vi "Butterfly_PullDown Capacitance _ERMod.vi"(0 "Semiconductor Module Context":T2, 1 "Capacitance":bool=TRUE, 3 "RFPins":string[](array[string]), 4 "VNAs Measurement Parameters":T1, 5 "error in (no error)":errorcluster, 7 "C_TH_Delta":dbl=2.0, 8 "R Thresholds":dbl[](array[numeric]), 9 "Start_v":dbl=10.0 format="%#_13g", 11 "Stop_v":dbl=41.0 format="%#_13g") -> (14 "Semiconductor Module Context Out":T2, 19 "error out":errorcluster)   [LabVIEW 2013]
uses:
  <vilib>/NI_TestStand_SemiconductorModule/NI_TestStand_Semiconductor_Module.lvlibp/PinMap/General/SemiconductorModuleContext.ctl
  VNA/VNAs Measurement Parameters.ctl
  <instrlib>/niDCPower/nidcpower.llb/niDCPower Wait For Event - Event.ctl
  <vilib>/NI_TestStand_SemiconductorModule/NI_TestStand_Semiconductor_Module.lvlibp/PinMap/DC Power/PinsToNIDCPowerSessions.vi
  <vilib>/NI_TestStand_SemiconductorModule/NI_TestStand_Semiconductor_Module.lvlibp/PinMap/General/Publish/PublishDataDoubleFunctionalTest.vi
  <vilib>/NI_TestStand_SemiconductorModule/NI_TestStand_Semiconductor_Module.lvlibp/PinMap/General/Publish/PublishDataDouble2D.vi
  <vilib>/NI_TestStand_SemiconductorModule/NI_TestStand_Semiconductor_Module.lvlibp
  VNA/Pin Map API/VNA Custom Instrument.lvlib
panel:
  out "C_Free":dbl[](array[numeric])
  out "VRLs":dbl[][](array[numeric]) format="%#_3g"
  out "VPIs":dbl[][](array[numeric]) format="%#_3g"
  out "appended array":dbl[][](array[numeric]) format="%#_3g"
  out "S3 steps":dbl[](array[numeric]) format="%#_3g"
  out "S2 steps":dbl[](array[numeric]) format="%#_3g"
  out "S1 steps":dbl[](array[numeric]) format="%#_3g"
  out "S0 steps":dbl[](array[numeric]) format="%#_3g"
  out "BF values":dbl[](array[numeric])
  out "VRLs":dbl[](array[numeric])
  out "VPIs":dbl[](array[numeric])
  out "Multisite Cap Data":dbl[][][](array[numeric])
  out "Full Array":dbl[][][](array[numeric])
  out "BF Names":string[](array[string])
  in  "current level":dbl=0.01 format="%_6p"
  out "R Array":dbl[](array[numeric])
  out "BFSamples":i32
  in  "Step_v":dbl=1.0
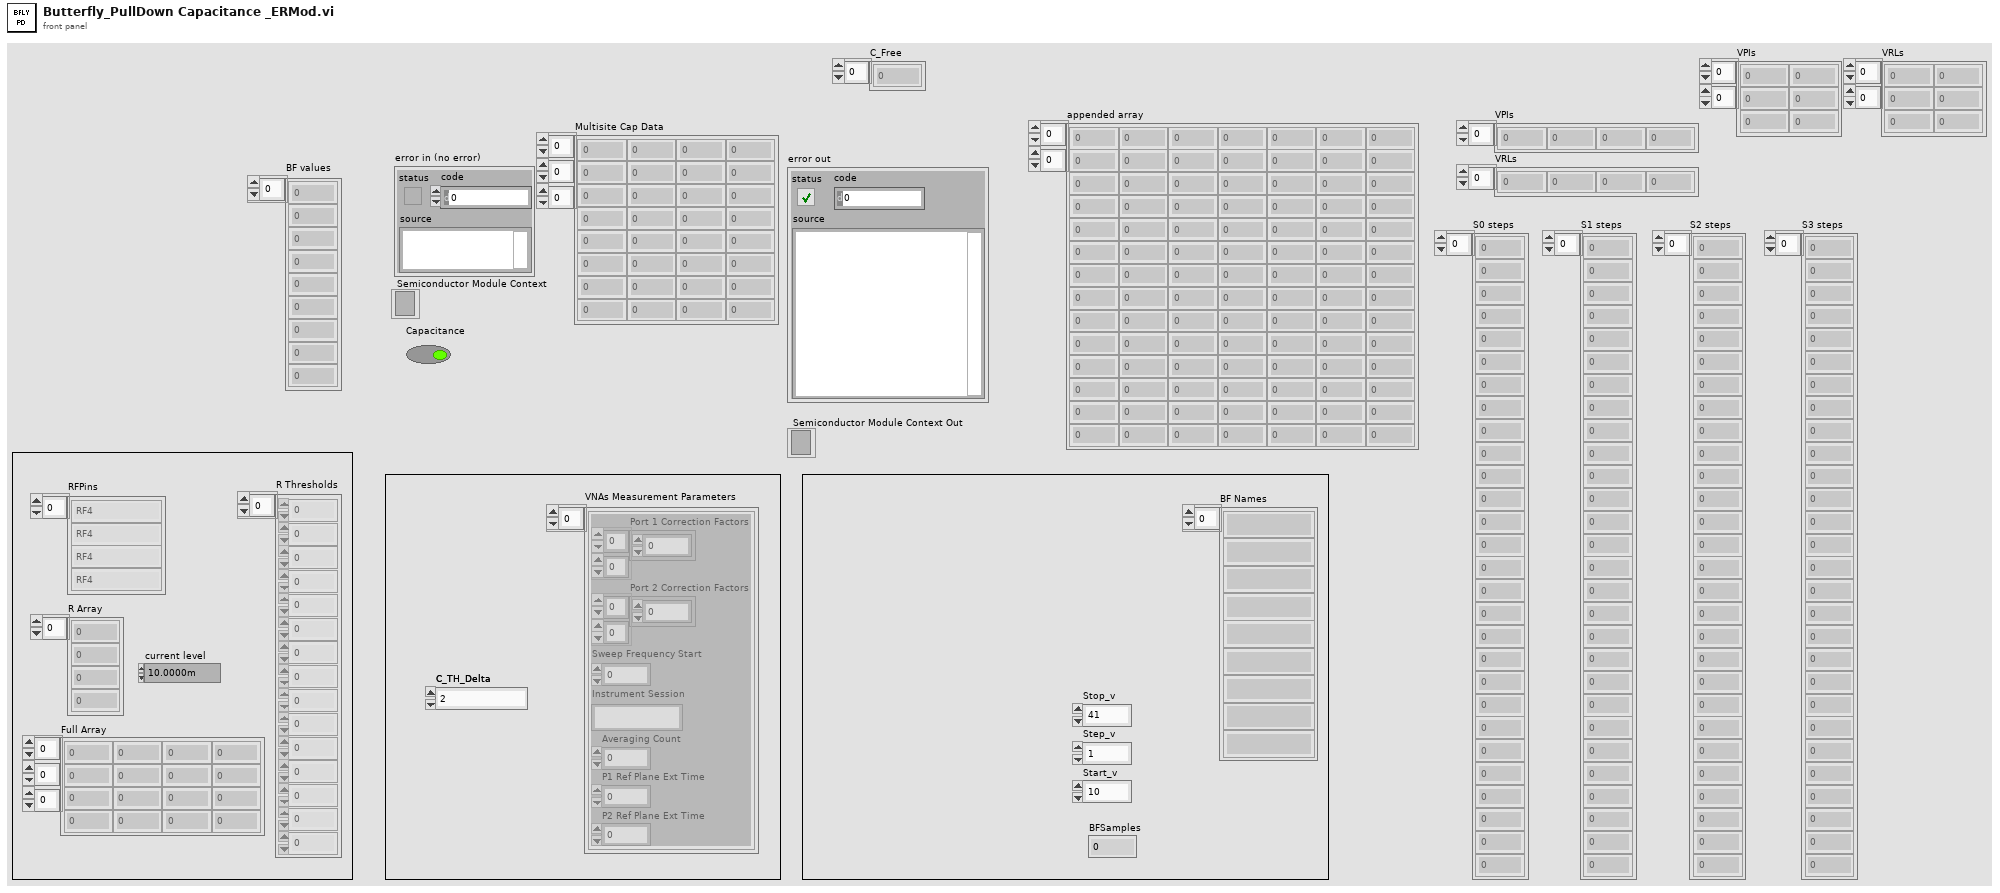
[diagram p1: front panel]
types:
  T1 = typedef "VNAs Measurement Parameters.ctl" = cluster{"Port 1 Correction Factors":cdb[][], "Port 2 Correction Factors":cdb[][], "Sweep Frequency Start":dbl, "Instrument Session":string, "Averaging Count":i32, "P1 Ref Plane Ext Time":dbl, "P2 Ref Plane Ext Time":dbl}[]
  T2 = typedef "NI_TestStand_Semiconductor_Module.lvlibp/SemiconductorModuleContext.ctl" = refnum<k7>
  T3 = typedef "niDCPower Wait For Event - Event.ctl" = i32
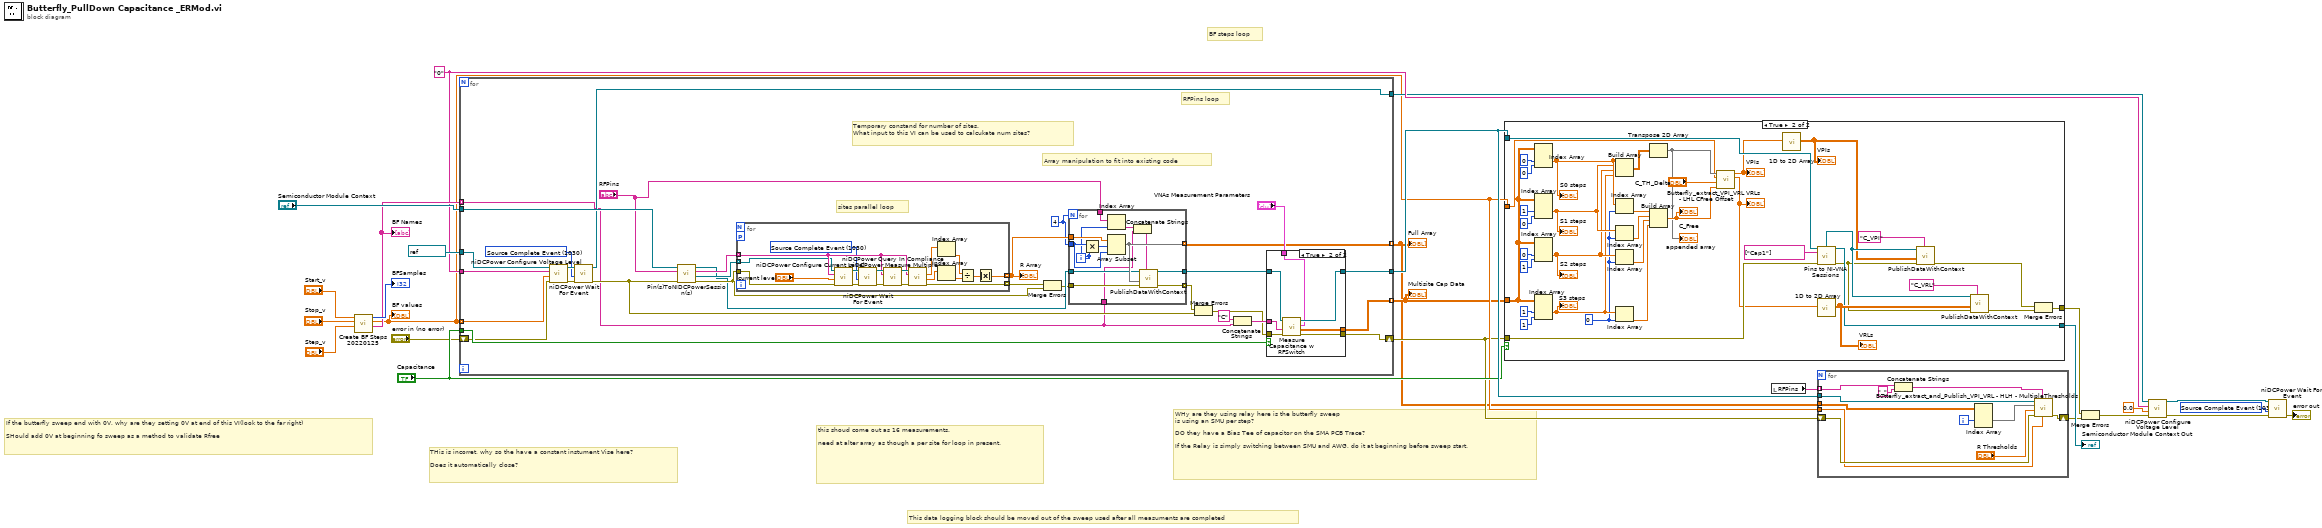
[diagram p0: block diagram]
diagram:
  w8 = T3 1030 items=["Source Complete Event"=1030, "Measure Complete Event"=1031, "Sequence Iteration Complete Event"=1032, "Sequence Engine Done Event"=1033, "Pulse Complete Event"=1051, "Ready For Pulse Trigger Event"=1052] ("event")
  w13 = "0" ("channel name")
  # "If the butterfly sweep end with 0V, why are they setting 0V at end of this VI(look to the far right)\n\nSHould add 0V at beginning fo sweep as a method to validate Rfree"
  # "This data logging block should be moved out of the sweep used after all measuments are completed"
  # "THis is incorret, why so the have a constant instument Vise here?\n\nDoes it automatically close?"
  # "WHy are they using relay here is the butterfly sweep \nis using an SMU per step?\n\nDO they have a Bias Tee of capacitor on the SMA PCB Trace?\n\nIf the Relay is simply switching between SMU and AWG, do it at beginning before sweep start."
  # "this shoud come out as 16 measurements. \n\nneed at alter array as though a per site for loop in present."
  # "BF steps loop"
  n1 = call "Create BF Steps 20220125.vi"("Step_v"="Step_v", "Stop_v"="Stop_v", "Start_v"="Start_v") -> ("BF Names"=w17:string[], "BF values"=w7:dbl[], "BFSamples"=→"BFSamples":i32)  [unwired: 6 in]
  "BF Names" <- w17
  "BF values" <- w7
  n2 = for {
    shift-right: [w40] -> w5
    shift-left: "error in (no error)" -> [w46]
    tunnel: "Semiconductor Module Context" -> [w57]
    tunnel: [w56] -> w23
    tunnel: [w52] -> w6 mode=indexing
    tunnel: "Capacitance" -> [w50]
    tunnel: w17 -> [w27] mode=indexing
    tunnel: w7 -> [w44] mode=indexing
    tunnel: w13 -> [w43]
    tunnel: refnum<k15> "4139_1" ("instrument handle") -> [w42]
    tunnel: [w41] -> w12
    tunnel: [w33] -> w1 mode=indexing
    w34 = 4
    w48 = T3 1030 items=["Source Complete Event"=1030, "Measure Complete Event"=1031, "Sequence Iteration Complete Event"=1032, "Sequence Engine Done Event"=1033, "Pulse Complete Event"=1051, "Ready For Pulse Trigger Event"=1052] ("event")
    # "Array manipulation to fit into existing code"
    # "Temporary constand for number of sites.\nWhat input to this VI can be used to calcukate num sites?"
    # "sites parallel loop"
    # "RFPins loop"
    n3 = call <instrlib>:"niDCPower Configure Voltage Level.vi"("error in (no error)"=w46, "voltage level"=w44, "channel name"=w43, "instrument handle"=w42) -> ("error out"=w47:errorcluster, "instrument handle out"=w49:refnum<k15>)  [unwired: 6 in]
    n4 = call <instrlib>:"niDCPower Wait For Event.vi"("error in (no error)"=w47, "event"=w48, "instrument handle"=w49) -> ("error out"=w45:errorcluster, "instrument handle out"=w41:refnum<k15>)  [unwired: 7 in]
    n5 = call-poly <vilib>:"Pin(s)ToNIDCPowerSession(s).vi"("error in (no error)"=w45, "Pins"="RFPins", "Semiconductor Module Context"=w57) -> ("error out"=w37:errorcluster, "Instrument Sessions"=w38:refnum<k15>[], "Channel Lists"=w39:string[], "Semiconductor Module Context Out"=w32:T2)  [unwired: 4 in, 1 out]
    n6 = for {
      tunnel: w39 -> [w75] mode=indexing
      tunnel: w38 -> [w71] mode=indexing
      tunnel: w37 -> [w72]
      tunnel: [w76] -> w35 mode=indexing
      workers-P: _ -> [_]
      tunnel: [w73] -> w36 mode=indexing
      w74 = T3 1030 items=["Source Complete Event"=1030, "Measure Complete Event"=1031, "Sequence Iteration Complete Event"=1032, "Sequence Engine Done Event"=1033, "Pulse Complete Event"=1051, "Ready For Pulse Trigger Event"=1052] ("event")
      n7 = call <instrlib>:"niDCPower Configure Current Level.vi"("error in (no error)"=w72, "current level"="current level", "channel name"=w75, "instrument handle"=w71) -> ("error out"=w84:errorcluster, "instrument handle out"=w83:refnum<k15>)  [unwired: 6 in]
      n8 = call <instrlib>:"niDCPower Wait For Event.vi"("error in (no error)"=w84, "event"=w74, "instrument handle"=w83) -> ("error out"=w88:errorcluster, "instrument handle out"=w87:refnum<k15>)  [unwired: 7 in]
      n9 = call <instrlib>:"niDCPower Query In Compliance.vi"("error in (no error)"=w88, "channel name"=w75, "instrument handle"=w87) -> ("error out"=w85:errorcluster, "instrument handle out"=w86:refnum<k15>)  [unwired: 6 in, 1 out]
      n10 = call <instrlib>:"niDCPower Measure Multiple.vi"("error in (no error)"=w85, "channel name"=w75, "instrument handle"=w86) -> ("error out"=w73:errorcluster, "current measurements"=w77:dbl[], "voltage measurements"=w78:dbl[])  [unwired: 5 in, 1 out]
      n11 = Index Array(array=w78) -> (element=w80:dbl)  [unwired: 1 in]
      n12 = Index Array(array=w77) -> (element=w79:dbl)  [unwired: 1 in]
      n13 = Divide(x=w80, y=w79) -> (x/y=w81:dbl)
      n14 = Absolute Value(x=w81) -> (abs(x)=w76:dbl)
    }
    "R Array" <- w35
    n15 = Merge Errors(w36, w37) -> (w30:errorcluster)
    n16 = for {
      N: w34 -> [_]
      tunnel: w35 -> [w70]
      tunnel: w34 -> [w69]
      tunnel: [w67] -> w33 mode=indexing
      tunnel: w32 -> [w66]
      tunnel: [w65] -> w31
      tunnel: w30 -> [w64]
      tunnel: [w63] -> w29 mode=indexing
      tunnel: "RFPins" -> [w62]
      tunnel: w27 -> [w60]
      i -> [w61]
      n17 = Multiply(x=w69, y=w61) -> (x*y=w68:i32)
      n18 = Array Subset(array=w70, index=w68, length=w69) -> (w67:dbl[])
      n19 = Index Array(array=w62, index=w61) -> (element=w59:string)
      n20 = Concatenate Strings(w59, w60) -> (w58:string)
      n21 = call-poly <vilib>:"PublishDataWithContext.vi"("Published Data Id"=w58, "error in (no error)"=w64, "Data In"=w67, "Semiconductor Module Context"=w66) -> ("error out"=w63:errorcluster, "Semiconductor Module Context Out"=w65:T2)  [unwired: 6 in]
    }
    n22 = Merge Errors(w29, w45) -> (w51:errorcluster)
    n23 = Concatenate Strings("C" ("string"), w27) -> (w54:string)
    n24 = case shown="True" w50 {
      tunnel: w31 -> [w90 w97]
      tunnel: [w90 w96] -> w56
      tunnel: [w89 w95] -> w40
      tunnel: w54 -> [_ w94]
      tunnel: "VNAs Measurement Parameters" -> [_ w93]
      tunnel: [_ w92] -> w52
      tunnel: w51 -> [w89 w91]
      frame False {
      }
      frame True {
        n25 = call "Measure Capacitance w RFSwitch.vi"("VNAs Measurement Parameters"=w93, "error in (no error)"=w91, "Measurement Id"=w94, "Semiconductor Module Context"=w97) -> ("error out"=w95:errorcluster, "Multisite Cap Data"=w92:dbl[][], "Semiconductor Module Context Out"=w96:T2)  [unwired: 5 in]
      }
    }
  }
  "Full Array" <- w1
  "Multisite Cap Data" <- w6
  n26 = case shown="True" "Capacitance" {
    tunnel: [w98 w118] -> w24
    tunnel: [w99 w136] -> w4
    tunnel: w23 -> [w98 w135]
    tunnel: w5 -> [w99 w131]
    tunnel: w7 -> [_ w103]
    tunnel: w6 -> [_ w122]
    frame False {
    }
    frame True {
      w111 = 0 ("index")
      n27 = Index Array(array=w122, index (dim 1)=0 ("disabled index (row)"), index (dim 2)=0 ("disabled index (col)")) -> (element=w115:dbl[])  [unwired: 1 in]
      "S0 steps" <- w115
      n28 = Index Array(array=w122, index (dim 1)=1 ("index (row)"), index (dim 2)=0 ("index (col)")) -> (element=w114:dbl[])  [unwired: 1 in]
      "S1 steps" <- w114
      n29 = Index Array(array=w122, index (dim 1)=0 ("index (row)"), index (dim 2)=1 ("index (col)")) -> (element=w113:dbl[])  [unwired: 1 in]
      "S2 steps" <- w113
      n30 = Index Array(array=w122, index (dim 1)=1 ("index (row)"), index (dim 2)=1 ("index (col)")) -> (element=w112:dbl[])  [unwired: 1 in]
      "S3 steps" <- w112
      n31 = Build Array(w115, w114, w113, w112) -> (w106:dbl[][])
      n32 = Index Array(array=w115, index=w111) -> (element=w110:dbl)
      n33 = Index Array(array=w114, index=w111) -> (element=w109:dbl)
      n34 = Index Array(array=w113, index=w111) -> (element=w108:dbl)
      n35 = Index Array(array=w112, index=w111) -> (element=w107:dbl)
      n36 = Transpose 2D Array(2D array=w106) -> (transposed array=w104:dbl[][])
      "appended array" <- w104
      n37 = Build Array(w110, w109, w108, w107) -> (w105:dbl[])
      "C_Free" <- w105
      n38 = call "Butterfly_extract_VPI_VRL - LHL CFree Offset.vi"("C_Free"=w105, "Delta"="C_TH_Delta", "Voltage Array"=w103, "Result Array In"=w104) -> ("VRLs"=w100:dbl[], "VPIs"=w101:dbl[])  [unwired: 6 in]
      "VPIs" <- w101
      "VRLs" <- w100
      n39 = call "1D to 2D Array.vi"("1D Array"=w101) -> ("2D Array"=w120:dbl[][])  [unwired: 10 in]
      "VPIs" <- w120
      n40 = call "Pins to NI-VNA Sessions.vi"("Semiconductor Module Context"=w135, "Pins"=string[] ["Cap1"] ("Capacitance Pins"), "error in (no error)"=w131) -> ("Pin Query Context"=w121:refnum<class "MultiplePinMultipleSessionQueryContext.lvclass">, "Semiconductor Module Context Out"=w118:T2, "error out"=w116:errorcluster)  [unwired: 8 in, 2 out]
      n41 = call "1D to 2D Array.vi"("1D Array"=w100) -> ("2D Array"=w134:dbl[][])  [unwired: 10 in]
      "VRLs" <- w134
      n42 = call-poly <vilib>:"PublishDataWithContext.vi"("Published Data Id"="C_VPI", "error in (no error)"=w116, "Data In"=w120, "Pin Query Context"=w121) -> ("error out"=w117:errorcluster)  [unwired: 6 in, 1 out]
      n43 = call-poly <vilib>:"PublishDataWithContext.vi"("Published Data Id"="C_VRL", "error in (no error)"=w116, "Data In"=w134, "Pin Query Context"=w121) -> ("error out"=w137:errorcluster)  [unwired: 6 in, 1 out]
      n44 = Merge Errors(w117, w137) -> (w136:errorcluster)
    }
  }
  "Semiconductor Module Context Out" <- w24
  n45 = local read "RFPins"() -> (w26:string[])
  n46 = for {
    tunnel: w26 -> [w144] mode=indexing
    shift-right: [w145] -> w3
    shift-left: w5 -> [w146]
    tunnel: w23 -> [w141]
    tunnel: w7 -> [w140]
    tunnel: w1 -> [w139]
    i -> [w148]
    n47 = Concatenate Strings(w144, "_" ("string")) -> (w142:string)
    n48 = Index Array(array=w139, index (dim 1)=w148) -> (element=w138:dbl[][])  [unwired: 2 in]
    n49 = call "Butterfly_extract_and_Publish_VPI_VRL - HLH - MultipleThresholds.vi"("Voltages Array"=w140, "ID Prefix"=w142, "error in (no error)"=w146, "Thresholds"="R Thresholds", "Result Array In"=w138, "Semiconductor Module Context"=w141) -> ("error out"=w145:errorcluster)  [unwired: 5 in]
  }
  n50 = Merge Errors(w4, w3) -> (w2:errorcluster)
  n51 = call <instrlib>:"niDCPower Configure Voltage Level.vi"("error in (no error)"=w2, "voltage level"=0.0, "channel name"=w13, "instrument handle"=w12) -> ("error out"=w11:errorcluster, "instrument handle out"=w9:refnum<k15>)  [unwired: 6 in]
  n52 = call <instrlib>:"niDCPower Wait For Event.vi"("error in (no error)"=w11, "event"=w8, "instrument handle"=w9) -> ("error out"=→"error out":errorcluster)  [unwired: 7 in, 1 out]
